vi "CTE_Analysis_Suite_InputMaker_FormatString.vi"(8 "VALUE":string, 11 "NAME":string) -> (3 "Output":string)   [LabVIEW 2012]
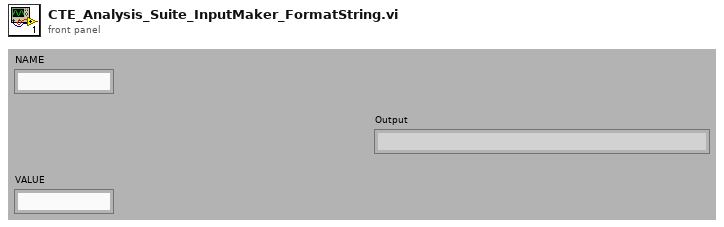
[diagram p1: front panel]
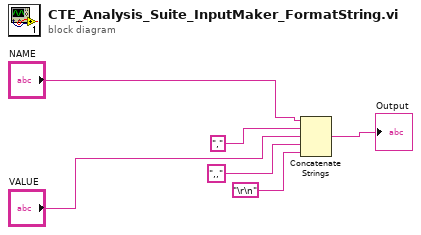
[diagram p0: block diagram]
diagram:
  n1 = Concatenate Strings("NAME", ",", "VALUE", ",,", "\r\n") -> (→"Output":string)
